vi "Error Codes File Window.vi"(5 "mode":T1 items=["create", "edit"], 7 "scope":T2=enum."global", 8 "error in (no error)":errorcluster, 10 "owner path":string, 11 "error list <top> in":variant) -> (0 "error out":errorcluster, 1 "cancelled?":bool, 2 "modified?":bool, 3 "error list <top> out":variant)   [LabVIEW 2017]
uses:
  Error List/Scope.ctl
  Controls/Error Code Window Modes.ctl
  Controls/Error Codes File Window Data.ctl
  Controls/Error Codes File Window States.ctl
  <vilib>/Utility/miscctls.llb/LVPointTypeDef.ctl
  Error File Management/Controls/NI Error.ctl
  Error List/Error Code File Properties.ctl
  Error File Management/Error File Management.lvlib
panel:
  out "frame name (create)":string="New Error Codes File"
  out "frame name (edit)":string="Error Codes File"
  out "owner":string caption="Owner File"
  in  "explore":bool
  in  "display name":string caption="Range Display Name (localized name that users will see in the Error Ring)"
  in  "family name":string caption="Range Name (non-localized name stored in the Error Ring)"
  in  "cancel":bool
  in  "ok":bool
  in  "comment":string caption="Comments about this file"
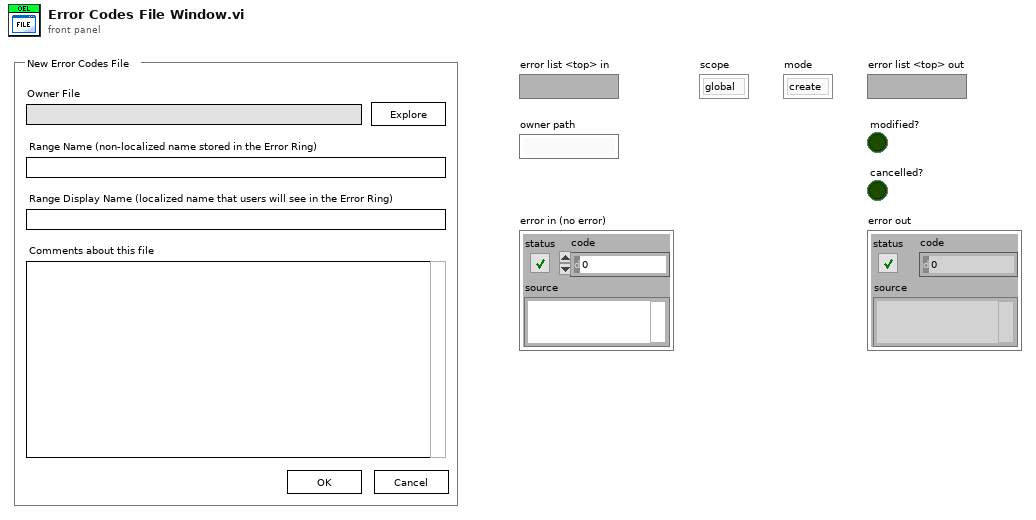
[diagram p1: front panel]
types:
  T1 = typedef "Error Code Window Modes.ctl" = u8
  T2 = typedef "Scope.ctl" = enum16{"project", "global"}
  T3 = typedef "Error Codes File Window States.ctl" = enum16{"init", "open FP", "idle", "modify", "close"}
  T4 = typedef "Error Codes File Window Data.ctl" = cluster{"mode":T1, "error list <top>":variant, "scope":T2, "owner":string, "owner path":path, "state":T3, "modified?":bool, "cancelled?":bool}
  T5 = typedef "LVPointTypeDef.ctl" = cluster{"Horizontal":i16, "Vertical":i16}
  T6 = typedef "Error Code File Properties.ctl" = cluster{"path":path, "simplified path":string, "name":string, "display name":string, "family name":string, "comment":string, "parsable?":bool, "file modified?":bool}
  T7 = typedef "Error File Management.lvlib/NI Error.ctl" = errorcluster
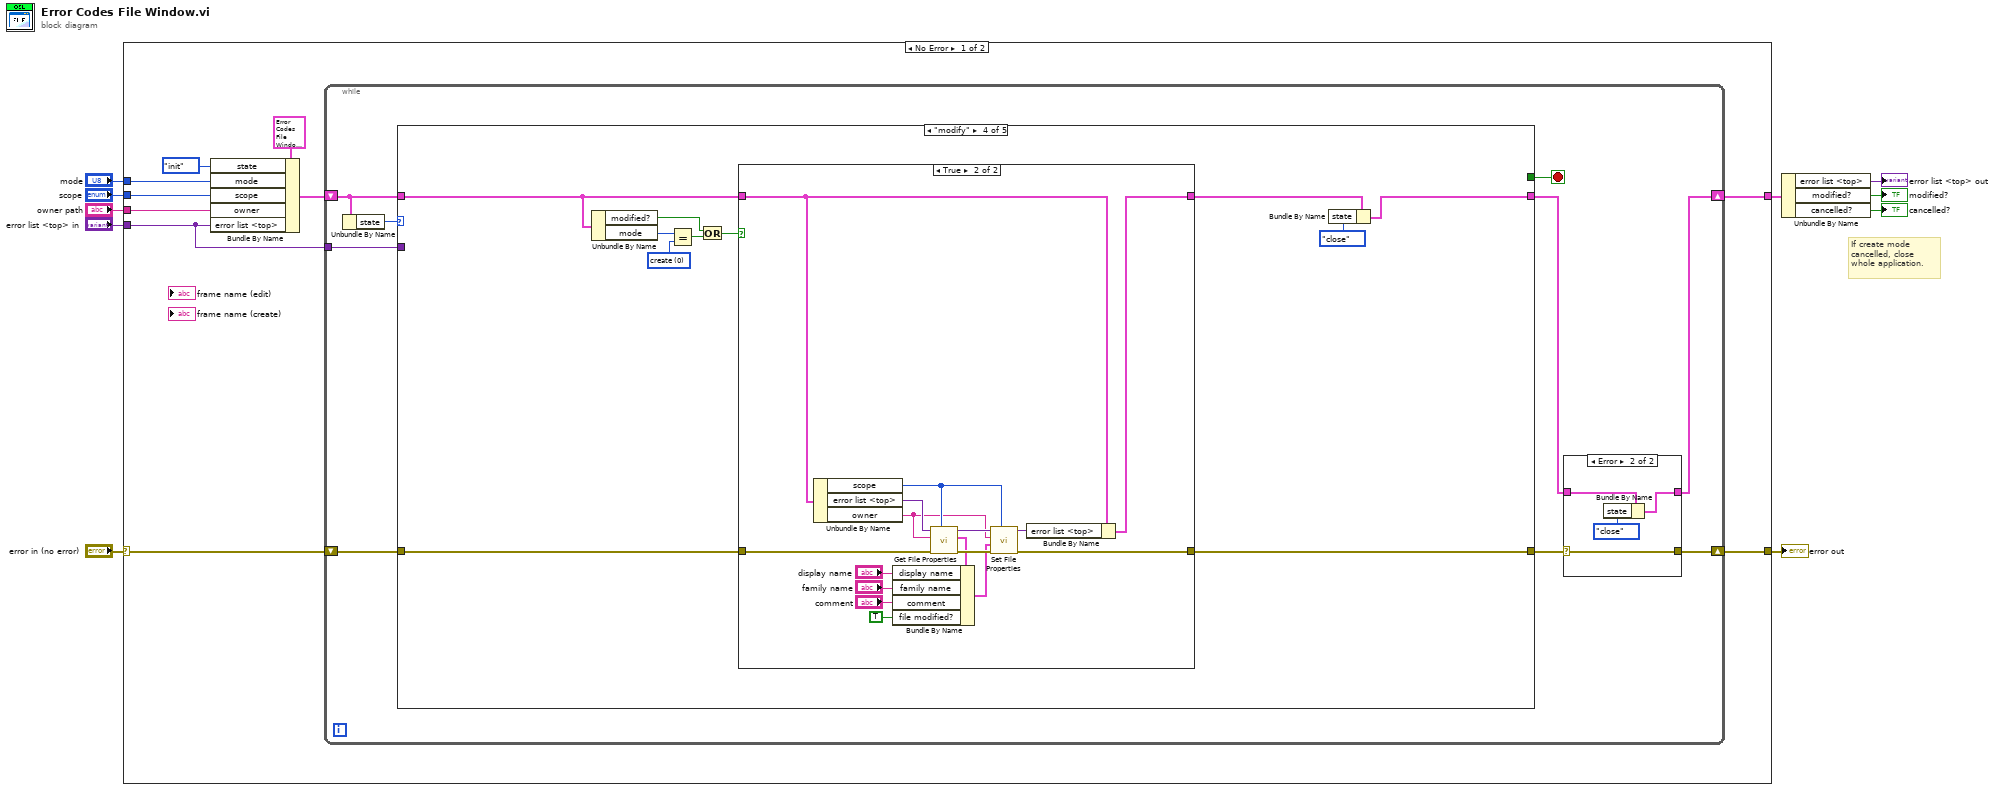
[diagram p0: block diagram]
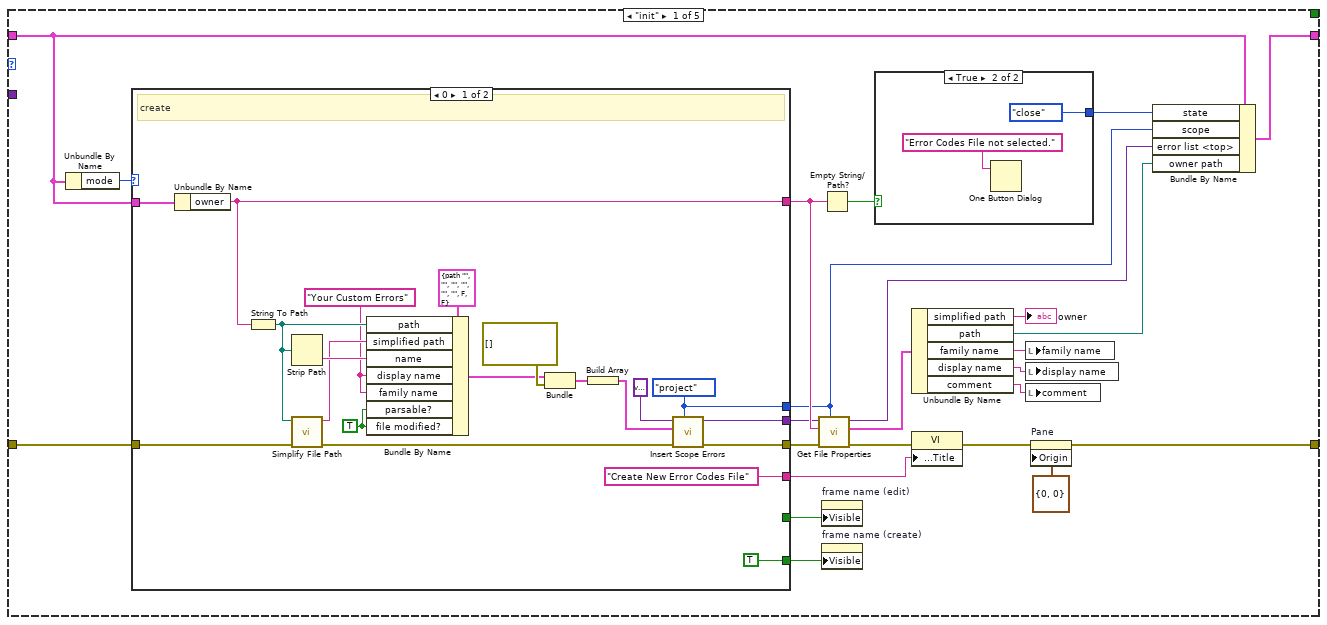
[diagram p3: hidden frame]
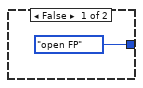
[diagram p4: hidden frame]
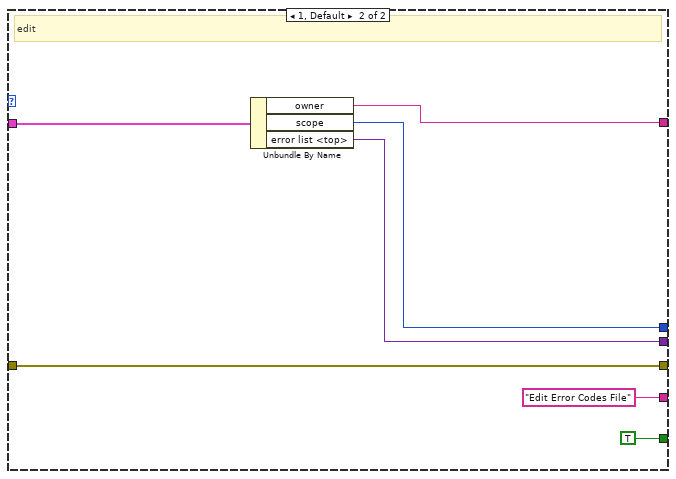
[diagram p5: hidden frame]
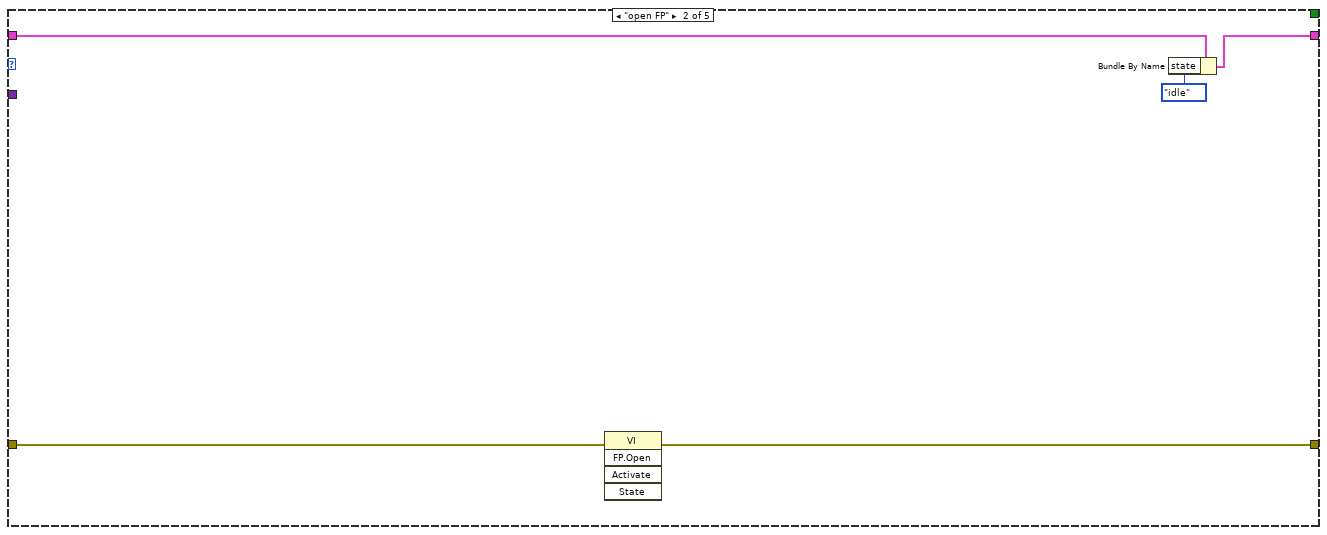
[diagram p6: hidden frame]
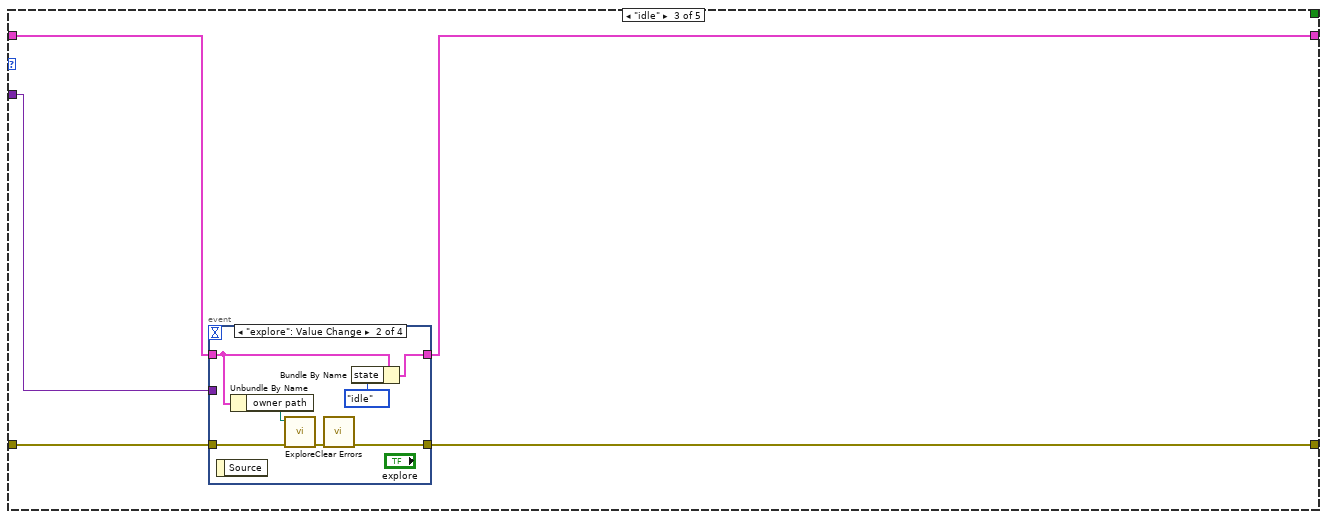
[diagram p7: hidden frame]
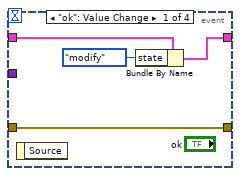
[diagram p8: hidden frame]
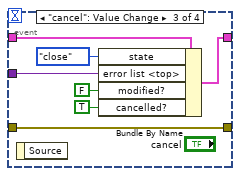
[diagram p9: hidden frame]
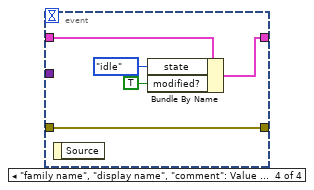
[diagram p10: hidden frame]
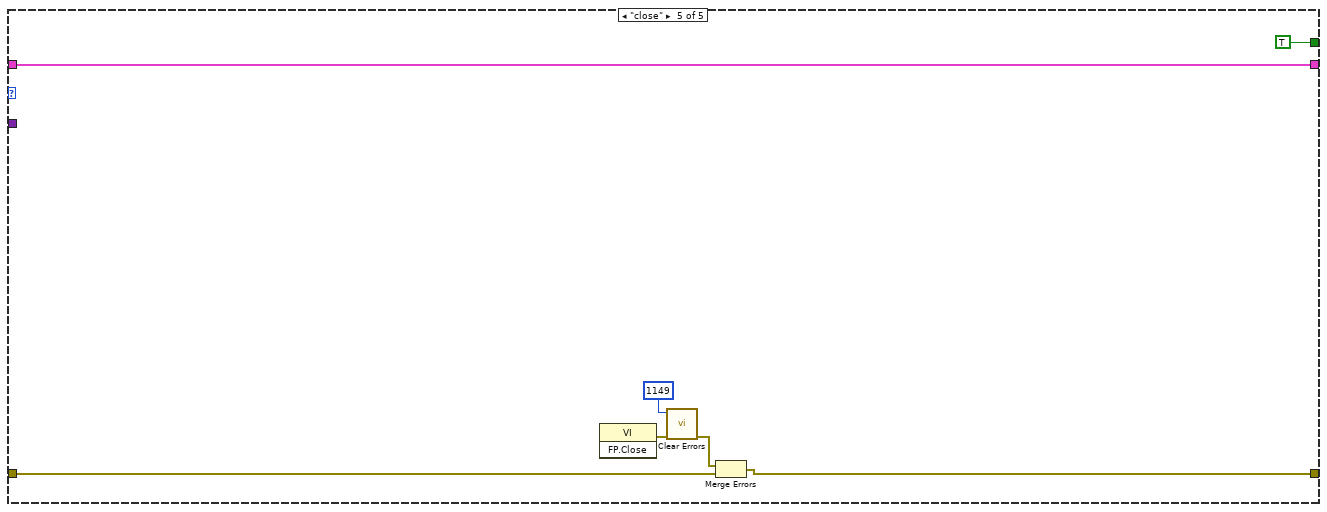
[diagram p12: hidden frame]
diagram:
  # "If create mode cancelled, close whole application."
  n1 = case shown="No Error" "error in (no error)" {
    selector: "error in (no error)" -> [w20 w159]
    tunnel: "mode" -> [w15 _]
    tunnel: "owner path" -> [w16 _]
    tunnel: "error list <top> in" -> [w13 _]
    tunnel: "scope" -> [w14 _]
    tunnel: [w12 w159] -> w5
    tunnel: [w11 _] -> w4
    frame No Error {
      n2 = Bundle By Name(cluster=T4 {"mode"=0, "error list <top>"=variant, "scope"=enum."project", "owner"="", "owner path"=path "", "state"=enum."modify", "modified?"=FALSE, "cancelled?"=FALSE} ("data"), "state"=Error_Codes_File_Window_States."init", "mode"=w15, "scope"=w14, "owner"=w16, "error list <top>"=w13) -> (w18:T4)
      n3 = while {
        shift-right: [w23] -> w12
        shift-left: w20 -> [w29]
        tunnel: w13 -> [w28]
        shift-right: [w21] -> w11
        shift-left: w18 -> [w27]
        stop <- w25 stop-if-true
        n4 = Unbundle By Name(w27) -> ("state"=w26:T3)
        n5 = case shown="\"modify\"" w26 {
          tunnel: w29 -> [w51 w91 w97 w133 w152]
          tunnel: [w46 w90 w96 w132 w153] -> w24
          tunnel: w28 -> [_ _ w95 _ _]
          tunnel: [w41 w92 w98 w124 w158] -> w22
          tunnel: w27 -> [w39 w93 w99 w126 w158]
          tunnel: [_ _ _ _ TRUE] -> w25
          frame "init" {
            n6 = Unbundle By Name(w39) -> ("mode"=w40:T1)
            n7 = case shown="0" w40 {
              tunnel: [w65 w86] -> w59
              tunnel: [w75 w85] -> w55
              tunnel: w51 -> [w73 w88]
              tunnel: [w71 w88] -> w50
              tunnel: [w68 w84] -> w42
              tunnel: ["Create New Error Codes File" "Edit Error Codes File"] -> w48
              tunnel: w39 -> [w66 w87]
              tunnel: [_ TRUE] -> w37
              tunnel: [TRUE _] -> w36
              frame 0 {
                w63 = "Your Custom Errors"
                w68 = Scope."project" ("scope")
                w69 = TRUE ("parsable?")
                # "create"
                n8 = Unbundle By Name(w66) -> ("owner"=w65:string)
                n9 = String To Path(string=w65) -> (path=w74:path)
                n10 = Strip Path(path=w74) -> (name=w77:string)  [unwired: 1 out]
                n11 = call "Simplify File Path.vi"("error in (no error)"=w73, "full path"=w74) -> ("error out"=w72:errorcluster, "simplified path"=w76:string)  [unwired: 8 in]
                n12 = Bundle By Name(cluster=T6 {"path"=path "", "simplified path"="", "name"="", "display name"="", "family name"="", "comment"="", "parsable?"=FALSE, "file modified?"=FALSE} ("properties"), "path"=w74, "simplified path"=w76, "name"=w77, "display name"=w63, "family name"=w63, "parsable?"=w69, "file modified?"=w69) -> (w78:T6)
                n13 = Bundle("properties"=w78, "errors"=T7[] []) -> (w81:cluster{"properties":T6, "errors":T7[]})  [unwired: 1 in]
                n14 = Build Array(w81) -> (w82:cluster{"properties":T6, "errors":T7[]}[])
                n15 = call "Insert Scope Errors.vi"("scope"=w68, "error in (no error)"=w72, "error codes file content"=w82, "error list <top> in"=variant) -> ("error out"=w71:errorcluster, "error list <top> out"=w75:variant)  [unwired: 6 in]
              }
              frame 1, Default {
                # "edit"
                n16 = Unbundle By Name(w87) -> ("owner"=w86:string, "scope"=w84:T2, "error list <top>"=w85:variant)
              }
            }
            n17 = call "Get File Properties.vi"("scope"=w42, "error in (no error)"=w50, "owner"=w59, "error list <top>"=w55) -> ("error out"=w49:errorcluster, "properties"=w57:T6, "error list <top> dup"=w43:variant)  [unwired: 5 in]
            n18 = Empty String/Path?(string/path=w59) -> (empty?=w45:bool)
            n19 = property on="frame name (edit)" class="Str"("Visible"=w37) -> ()  [unwired: 2 in, 2 out]
            n20 = property on="frame name (create)" class="Str"("Visible"=w36) -> ()  [unwired: 2 in, 2 out]
            n21 = case shown="True" w45 {
              tunnel: [Error_Codes_File_Window_States."open FP" Error_Codes_File_Window_States."close"] -> w38
              frame False {
              }
              frame True {
                n22 = One Button Dialog(message="Error Codes File not selected.") -> ()  [unwired: 1 in, 1 out]
              }
            }
            n23 = Unbundle By Name(w57) -> ("simplified path"=→"owner":string, "path"=w44:path, "family name"=w54:string, "display name"=w52:string, "comment"=w53:string)
            n24 = property class="VI"(error in=w49, "Front Panel.Title"=w48) -> (error out=w47:errorcluster)  [unwired: 1 in, 1 out]
            n25 = local write "family name"(w54) -> ()
            n26 = local write "display name"(w52) -> ()
            n27 = local write "comment"(w53) -> ()
            n28 = property on="Pane" class="Pane"(error in=w47, "Origin"=T5 {"Horizontal"=0, "Vertical"=0}) -> (error out=w46:errorcluster)  [unwired: 1 in, 1 out]
            n29 = Bundle By Name(cluster=w39, "state"=w38, "scope"=w42, "error list <top>"=w43, "owner path"=w44) -> (w41:T4)
          }
          frame "open FP" {
            n30 = invoke class="VI" method="FP.Open"(error in=w91) -> (error out=w90:errorcluster)  [unwired: 4 in, 4 out]
            n31 = Bundle By Name(cluster=w93, "state"=Error_Codes_File_Window_States."idle") -> (w92:T4)
          }
          frame "idle" {
            n32 = event shown="[1] \"explore\": Value Change" {
              selector: _ -> [_ _ _ _]
              dyn-events: _ -> [_ _ _ _]
              timeout: _ -> [_ _ _ _]
              tunnel: w99 -> [w103 w109 w117 w121]
              tunnel: [w102 w105 w116 w120] -> w98
              tunnel: w97 -> [w100 w107 w115 w122]
              tunnel: [w100 w106 w115 w122] -> w96
              tunnel: w95 -> [_ _ w114 _]
              event "ok": Value Change {
                n33 = event-data() -> ()  [unwired: 1 in, 1 out]
                n34 = Bundle By Name(cluster=w103, "state"=Error_Codes_File_Window_States."modify") -> (w102:T4)
              }
              event "explore": Value Change {
                n35 = event-data() -> ()  [unwired: 1 in, 1 out]
                n36 = Unbundle By Name(w109) -> ("owner path"=w108:path)
                n37 = call "Explore.vi"("error in (no error)"=w107, "file path"=w108) -> ("error out"=w110:errorcluster)  [unwired: 9 in]
                n38 = call <vilib>:"Clear Errors.vi"("error in (no error)"=w110) -> ("error out"=w106:errorcluster)  [unwired: 5 in, 1 out]
                n39 = Bundle By Name(cluster=w109, "state"=Error_Codes_File_Window_States."idle") -> (w105:T4)
              }
              event "cancel": Value Change {
                n40 = event-data() -> ()  [unwired: 1 in, 1 out]
                n41 = Bundle By Name(cluster=w117, "state"=Error_Codes_File_Window_States."close", "error list <top>"=w114, "modified?"=FALSE, "cancelled?"=TRUE) -> (w116:T4)
              }
              event "family name", "display name", "comment": Value Change {
                n42 = event-data() -> ()  [unwired: 1 in, 1 out]
                n43 = Bundle By Name(cluster=w121, "state"=Error_Codes_File_Window_States."idle", "modified?"=TRUE) -> (w120:T4)
              }
            }
          }
          frame "modify" {
            w130 = T1 0 items=["create", "edit"] ("y")
            n44 = Unbundle By Name(w126) -> ("modified?"=w128:bool, "mode"=w131:T1)
            n45 = Equal?(x=w131, y=w130) -> (x = y?=w129:bool)
            n46 = Or(x=w128, y=w129) -> (x .or. y?=w127:bool)
            n47 = case shown="True" w127 {
              tunnel: w126 -> [w134 w141]
              tunnel: w133 -> [w135 w138]
              tunnel: [w135 w137] -> w132
              tunnel: [w134 w136] -> w125
              frame False {
              }
              frame True {
                n48 = Unbundle By Name(w141) -> ("scope"=w143:T2, "error list <top>"=w142:variant, "owner"=w139:string)
                n49 = call "Get File Properties.vi"("scope"=w143, "error in (no error)"=w138, "owner"=w139, "error list <top>"=w142) -> ("error out"=w151:errorcluster, "properties"=w150:T6, "error list <top> dup"=w144:variant)  [unwired: 5 in]
                n50 = Bundle By Name(cluster=w150, "display name"="display name", "family name"="family name", "comment"="comment", "file modified?"=TRUE) -> (w149:T6)
                n51 = call "Set File Properties.vi"("scope"=w143, "error in (no error)"=w151, "properties"=w149, "owner"=w139, "error list <top>"=w144) -> ("error out"=w137:errorcluster, "error list <top> out"=w140:variant)  [unwired: 5 in]
                n52 = Bundle By Name(cluster=w141, "error list <top>"=w140) -> (w136:T4)
              }
            }
            n53 = Bundle By Name(cluster=w125, "state"=Error_Codes_File_Window_States."close") -> (w124:T4)
          }
          frame "close" {
            n54 = invoke class="VI" method="FP.Close"() -> (error out=w156:errorcluster)  [unwired: 3 in, 2 out]
            n55 = call <vilib>:"Clear Errors.vi"("error in (no error)"=w156, "specific error code to clear (0: all)"=1149) -> ("error out"=w155:errorcluster)  [unwired: 4 in, 1 out]
            n56 = Merge Errors(w155, w152) -> (w153:errorcluster)
          }
        }
        n57 = case shown="Error" w24 {
          selector: w24 -> [w31 w33]
          tunnel: [w31 w33] -> w23
          tunnel: w22 -> [w30 w35]
          tunnel: [w30 w34] -> w21
          frame No Error {
          }
          frame Error {
            n58 = Bundle By Name(cluster=w35, "state"=Error_Codes_File_Window_States."close") -> (w34:T4)
          }
        }
      }
    }
    frame Error {
    }
  }
  "error out" <- w5
  n59 = Unbundle By Name(w4) -> ("error list <top>"=→"error list <top> out":variant, "modified?"=→"modified?":bool, "cancelled?"=→"cancelled?":bool)
